vi "Open a Document on Disk.vi"(4 "error in (no error)":errorcluster, 7 "document path":path) -> (0 "error out":errorcluster)   [LabVIEW 2020]
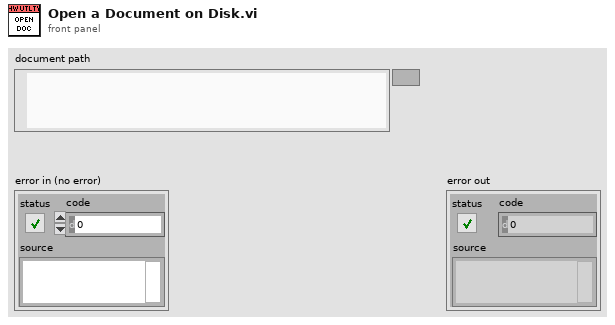
[diagram p1: front panel]
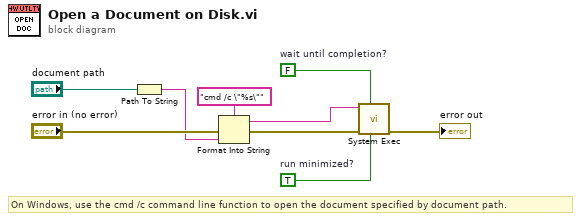
[diagram p0: block diagram]
diagram:
  w4 = TRUE  # run minimized?
  w8 = FALSE  # wait until completion?
  # "On Windows, use the cmd /c command line function to open the document specified by document path."
  n1 = Path To String(path="document path") -> (string=w2:string)
  n2 = Format Into String(format string="cmd /c \"%s\"", error in="error in (no error)", w2) -> (resulting string=w6:string, error out=w5:errorcluster)  [unwired: 1 in]
  n3 = call <vilib>:"System Exec.vi"("run minimized? (F)"=w4, "wait until completion? (T)"=w8, "error in (no error)"=w5, "command line"=w6) -> ("error out"=→"error out":errorcluster)  [unwired: 4 in, 3 out]
